vi "CreateUserEvents.vi"(8 "error in (no error)":errorcluster, 11 "UserEvents":T1) -> (0 "error out":errorcluster, 3 "UserEvents out":T1)   [LabVIEW 2022 SP3, in "Motor Controller.lvclass"]
uses:
  Motor Controller.lvclass
  Typedefs/UserEvents.ctl
  Typedefs/API Event Data.ctl
  Typedefs/API Task State.ctl
  Typedefs/Status.ctl
  TopLevel/Typedefs/Motor Controller Config Data.ctl
  Typedefs/Stage Move Data.ctl
  Typedefs/Batch Index Speed Data.ctl
  Typedefs/Move Status.ctl
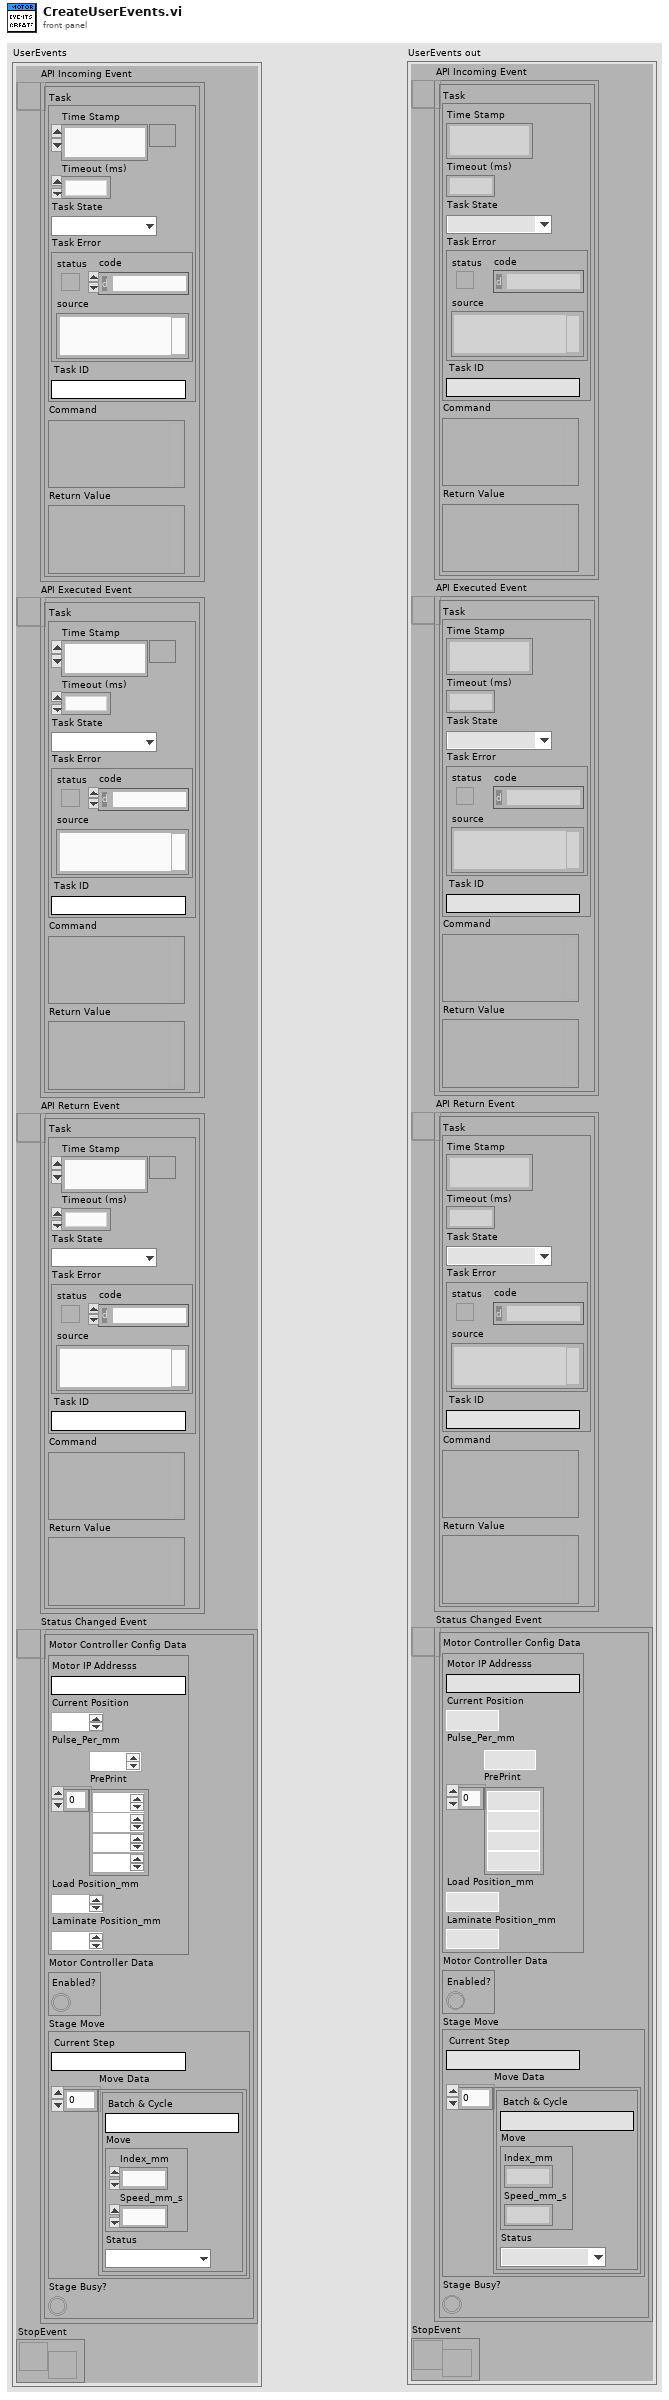
[diagram p1: front panel]
types:
  T1 = typedef "Motor Controller.lvclass/UserEvents.ctl" = cluster{"API Incoming Event":refnum<user-event>, "API Executed Event":refnum<user-event>, "API Return Event":refnum<user-event>, "Status Changed Event":refnum<user-event>, "StopEvent":refnum<user-event>}
  T2 = typedef "Motor Controller.lvclass/Status.ctl" = cluster{"Motor Controller Config Data":T3, "Motor Controller Data":cluster{"Enabled?":bool}, "Stage Move":T4, "Stage Busy?":bool}
  T3 = typedef "Motor Controller.lvclass/Motor Controller Config Data.ctl" = cluster{"Motor IP Addresss":string, "Current Position":i32, "Pulse_Per_mm":i32, "PrePrint":dbl[], "Load Position_mm":i32, "Laminate Position_mm":i32}
  T4 = typedef "Motor Controller.lvclass/Stage Move Data.ctl" = cluster{"Current Step":string, "Move Data":T5[]}
  T5 = typedef "Motor Controller.lvclass/Batch Index Speed Data.ctl" = cluster{"Batch & Cycle":string, "Move":cluster{"Index_mm":i32, "Speed_mm_s":i32}, "Status":T6}
  T6 = typedef "Motor Controller.lvclass/Move Status.ctl" = enum16{"Pending", "In Progress", "Completed"}
  T7 = typedef "Motor Controller.lvclass/API Event Data.ctl" = cluster{"Task":cluster{"Time Stamp":timestamp, "Timeout (ms)":u32, "Task State":T8, "Task Error":errorcluster, "Task ID":string}, "Command":variant, "Return Value":variant}
  T8 = typedef "Motor Controller.lvclass/API Task State.ctl" = enum16{"Completed", "Errored", "Pending"}
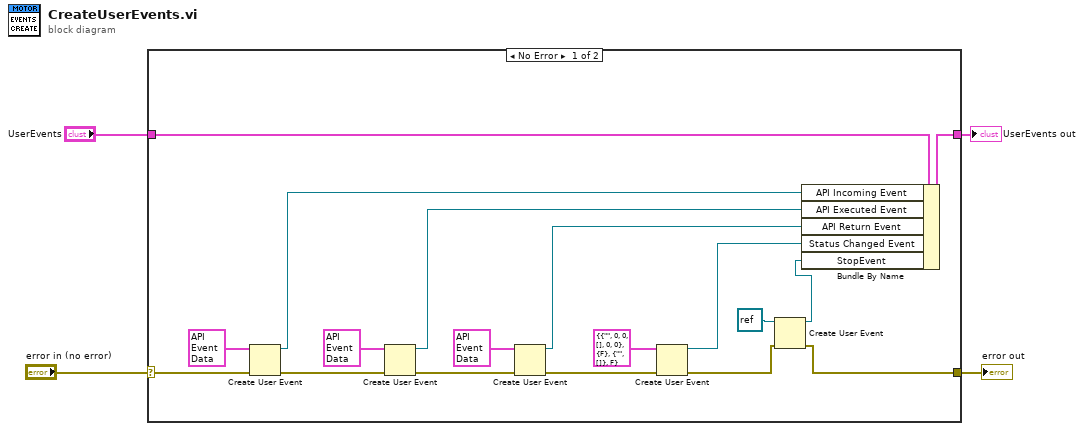
[diagram p0: block diagram]
diagram:
  n1 = case shown="No Error" "error in (no error)" {
    selector: "error in (no error)" -> [w18 w24]
    tunnel: [w6 w24] -> w3
    tunnel: "UserEvents" -> [w22 w23]
    tunnel: [w21 w23] -> w1
    frame No Error {
      n2 = Create User Event(user event datatype=T7 {"Task"={"Time Stamp"=timestamp(0 s since 1904-01-01), "Timeout (ms)"=0, "Task State"=enum."Completed", "Task Error"={"status"=FALSE, "code"=0, "source"=""}, "Task ID"=""}, "Command"=variant(enum16{"Event 1"} enum."Event 1"), "Return Value"=variant(string "")} ("API Event Data"), error in=w18) -> (user event=w19:refnum<user-event>, error out=w16:errorcluster)
      n3 = Create User Event(user event datatype=T7 {"Task"={"Time Stamp"=timestamp(0 s since 1904-01-01), "Timeout (ms)"=0, "Task State"=enum."Completed", "Task Error"={"status"=FALSE, "code"=0, "source"=""}, "Task ID"=""}, "Command"=variant(enum16{"Event 1"} enum."Event 1"), "Return Value"=variant(string "")} ("API Event Data"), error in=w16) -> (user event=w15:refnum<user-event>, error out=w13:errorcluster)
      n4 = Create User Event(user event datatype=T7 {"Task"={"Time Stamp"=timestamp(0 s since 1904-01-01), "Timeout (ms)"=0, "Task State"=enum."Completed", "Task Error"={"status"=FALSE, "code"=0, "source"=""}, "Task ID"=""}, "Command"=variant(enum16{"Event 1"} enum."Event 1"), "Return Value"=variant(string "")} ("API Event Data"), error in=w13) -> (user event=w12:refnum<user-event>, error out=w9:errorcluster)
      n5 = Create User Event(user event datatype=T2 {"Motor Controller Config Data"={"Motor IP Addresss"="", "Current Position"=0, "Pulse_Per_mm"=0, "PrePrint"=[], "Load Position_mm"=0, "Laminate Position_mm"=0}, "Motor Controller Data"={"Enabled?"=FALSE}, "Stage Move"={"Current Step"="", "Move Data"=[]}, "Stage Busy?"=FALSE} ("Status"), error in=w9) -> (user event=w10:refnum<user-event>, error out=w7:errorcluster)
      n6 = Create User Event(user event datatype=refnum<notifier> refnum ("notifier out"), error in=w7) -> (user event=w5:refnum<user-event>, error out=w6:errorcluster)
      n7 = Bundle By Name(cluster=w22, "API Incoming Event"=w19, "API Executed Event"=w15, "API Return Event"=w12, "Status Changed Event"=w10, "StopEvent"=w5) -> (w21:T1)
    }
    frame Error {
    }
  }
  "error out" <- w3
  "UserEvents out" <- w1
